vi "Real A x B (Optimized).vi"(2 "B":T1, 3 "A":T1) -> (0 "error":i32, 1 "A x B":T1)   [LabVIEW 2020, in "NI_AALBase.lvlib"]
uses:
  NI_AALBase.lvlib
  RealMatrix.ctl
  <resource>/lvanlys.dll
  NI_Matrix.lvlib
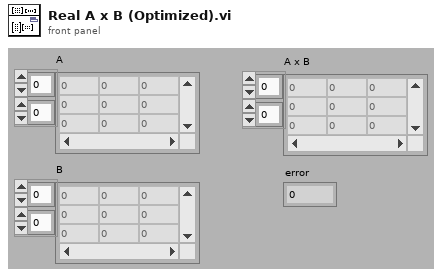
[diagram p1: front panel]
types:
  T1 = typedef "NI_Matrix.lvlib/RealMatrix.ctl" = dbl[][]
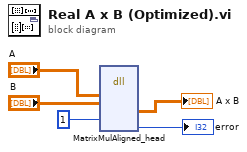
[diagram p0: block diagram]
diagram:
  n1 = dll-call lib="C:/Program Files (x86)/National Instruments/LabVIEW 2020/resource/lvanlys.*" fn="MatrixMulAligned_head"("aHandle"="A", "bHandle"="B", "isAligned"=1) -> ("cHandle"=→"A x B":dbl[][], "dsperr"=→"error":i32)  [unwired: 9 in, 2 out]
